vi "Waveform Attribute, Set DBL Reference.vi"(5 "Digital DBL Refnum":refnum<vi>, 6 "error in":errorcluster, 9 "waveform":waveform(dbl)) -> (0 "error out":errorcluster, 3 "waveform out":waveform(dbl))   [LabVIEW 2010]
doc: "Writes a array of Digital double precision (DBL) values as waveform attributes using a control references."
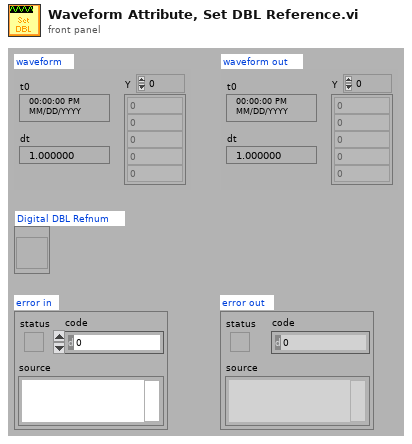
[diagram p1: front panel]
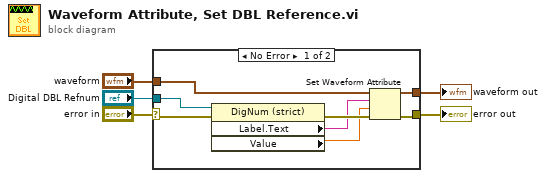
[diagram p0: block diagram]
diagram:
  n1 = case shown="No Error" "error in" {
    selector: "error in" -> [w12 w15]
    tunnel: [w13 w15] -> w5
    tunnel: "waveform" -> [w11 w14]
    tunnel: [w10 w14] -> w2
    tunnel: "Digital DBL Refnum" -> [w6 _]
    frame No Error {
      n2 = property class="DigNum (strict)"(reference=w6, error in=w12) -> (error out=w9:errorcluster, "Label.Text"=w7:string, "Value"=w8:dbl)  [unwired: 1 out]
      n3 = Set Waveform Attribute(4:w9, 5:w8, 6:w7, 7:w11) -> (0:w13:errorcluster, 3:w10:waveform(dbl))  [unwired: 1 out]
    }
    frame Error {
    }
  }
  "error out" <- w5
  "waveform out" <- w2
